vi "打开多模板.vi"(9 "原始记录模板":string, 11 "被测通道数":i32) -> (0 "错误输出":errorcluster, 3 "数组":refnum<class "NI_report.lvclass">[](array[class]))   [LabVIEW 2015]
uses:
  <vilib>/Utility/NIReport.llb/NI_report.lvclass
  Global.vi
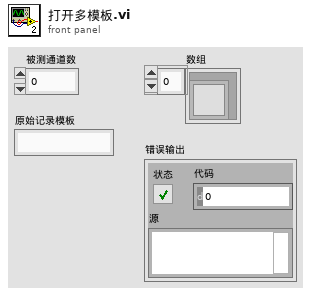
[diagram p1: front panel]
types:
  T1 = enum16{"Standard Report", "HTML", "Word", "Excel"}
  T2 = enum16{"maximized", "minimized", "normal", "no change"}
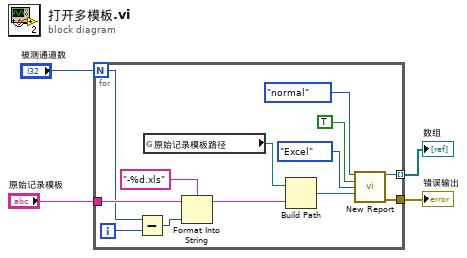
[diagram p0: block diagram]
diagram:
  n1 = for {
    N: "被测通道数" -> [w7]
    tunnel: [w12] -> w1
    tunnel: [w11] -> w3 mode=indexing
    tunnel: "原始记录模板" -> [w8]
    i -> [w6]
    n2 = Subtract(x=w7, y=w6) -> (x-y=w5:i32)
    n3 = global read "Global.vi" "原始记录模板路径"() -> (w17:path)
    n4 = Format Into String(format string="-%d.xls" ("字符串"), initial string=w8, w5) -> (resulting string=w9:string)  [unwired: 1 in, 1 out]
    n5 = Build Path(base path=w17, name or relative path=w9) -> (appended path=w13:path)
    n6 = call <vilib>:"New Report.vi"("window state (normal)"=T2."normal", "display alerts? (F)"=TRUE, "report type"=T1."Excel", "template (empty)"=w13) -> ("report out"=w11:refnum<class "NI_report.lvclass">, "error out"=w12:errorcluster)  [unwired: 10 in]
  }
  "数组" <- w3
  "错误输出" <- w1
